vi "AlarmData_to_Waveform_Arry.vi"(9 "dt":dbl=1.0 format="%#_13g", 10 "t0":timestamp, 11 "AI_channel_data":dbl[][](array[numeric])) -> (3 "Array":waveform(dbl)[](array[waveform]))   [LabVIEW 2018]
doc: "Format the 2D array of Alarm datapoints into an array of waveforms, suitable for display.\nOne waveform per Alarm channel."
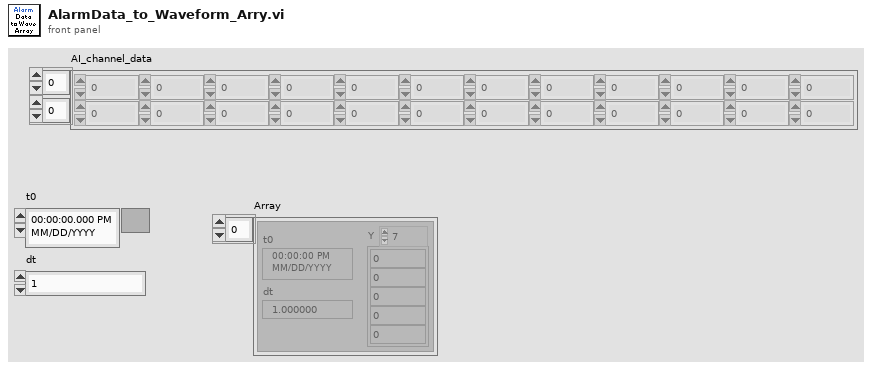
[diagram p1: front panel]
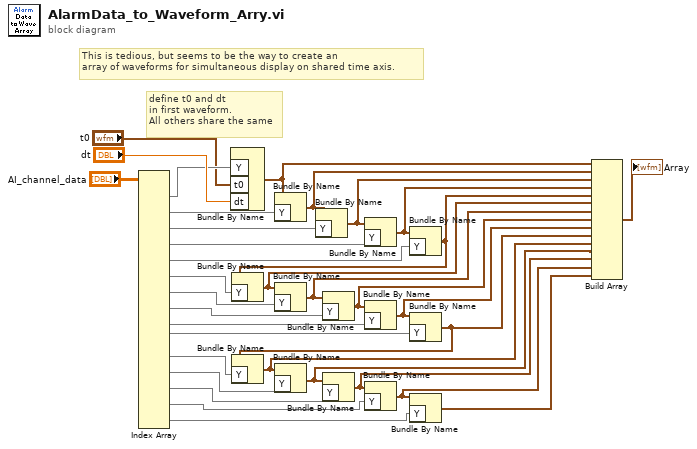
[diagram p0: block diagram]
diagram:
  # "define t0 and dt\nin first waveform.\nAll others share the same"
  # "This is tedious, but seems to be the way to create an\narray of waveforms for simultaneous display on shared time axis."
  n1 = Index Array(array="AI_channel_data") -> (element #1=w30:dbl[], element #2=w31:dbl[], element #3=w26:dbl[], element #4=w23:dbl[], element #5=w22:dbl[], element #6=w20:dbl[], element #7=w18:dbl[], element #8=w16:dbl[], element #9=w15:dbl[], element #10=w14:dbl[], element #11=w11:dbl[], element #12=w9:dbl[], element #13=w8:dbl[], element #14=w7:dbl[], element #15=w6:dbl[])  [unwired: 30 in]
  n2 = Bundle By Name("Y"=w30, "t0"="t0", "dt"="dt") -> (w32:waveform(dbl))  [unwired: 1 in]
  n3 = Bundle By Name(cluster=w32, "Y"=w31) -> (w27:waveform(dbl))
  n4 = Bundle By Name(cluster=w27, "Y"=w26) -> (w25:waveform(dbl))
  n5 = Bundle By Name(cluster=w25, "Y"=w23) -> (w24:waveform(dbl))
  n6 = Bundle By Name(cluster=w24, "Y"=w22) -> (w21:waveform(dbl))
  n7 = Bundle By Name(cluster=w21, "Y"=w20) -> (w19:waveform(dbl))
  n8 = Bundle By Name(cluster=w19, "Y"=w18) -> (w17:waveform(dbl))
  n9 = Bundle By Name(cluster=w17, "Y"=w16) -> (w13:waveform(dbl))
  n10 = Bundle By Name(cluster=w13, "Y"=w15) -> (w12:waveform(dbl))
  n11 = Bundle By Name(cluster=w12, "Y"=w14) -> (w10:waveform(dbl))
  n12 = Bundle By Name(cluster=w10, "Y"=w11) -> (w5:waveform(dbl))
  n13 = Bundle By Name(cluster=w5, "Y"=w9) -> (w4:waveform(dbl))
  n14 = Bundle By Name(cluster=w4, "Y"=w8) -> (w3:waveform(dbl))
  n15 = Bundle By Name(cluster=w3, "Y"=w7) -> (w2:waveform(dbl))
  n16 = Bundle By Name(cluster=w2, "Y"=w6) -> (w1:waveform(dbl))
  n17 = Build Array(w32, w27, w25, w24, w21, w19, w17, w13, w12, w10, w5, w4, w3, w2, w1) -> (→"Array":waveform(dbl)[])
